vi "Plane.SetLongitude.vi"(8 "error in (no error)":errorcluster, 10 "SetLongitude":T1, 11 "Plane":refnum<class "Plane.lvclass">) -> (0 "error out":errorcluster, 3 "Plane out":refnum<class "Plane.lvclass">)   [LabVIEW 2020, in "Plane.lvclass"]
doc: "---------------------------------------------------------------\nJKI State Machine Objects™\nhttp://jki.net/state-machine-objects/\nCopyright (C) 2005-2015, JKI <info@jki.net>\nALL RIGHTS RESERVEDJKI State Machine Objects (SMO) 1.0.0.4\nJKI - JKI\nCopyright (c) 2015, JKI"
uses:
  Plane.lvclass
  Plane.lvclass/Plane.ctl
  Typedefs/PrivateEvents--Plane.SetLongitude.ctl
panel:
  # "For instructions on how to use the JKI State Machine Objects, examples and video tutorials, visit:\nhttp://jki.net/state-machine-objects/\n\nJKI State Machine Objects™\nhttp://jki.net/state-machine-objects/\nCopyright (C) 2005-2015, JKI <info@jki.net>\nALL RIGHTS RESERVED"
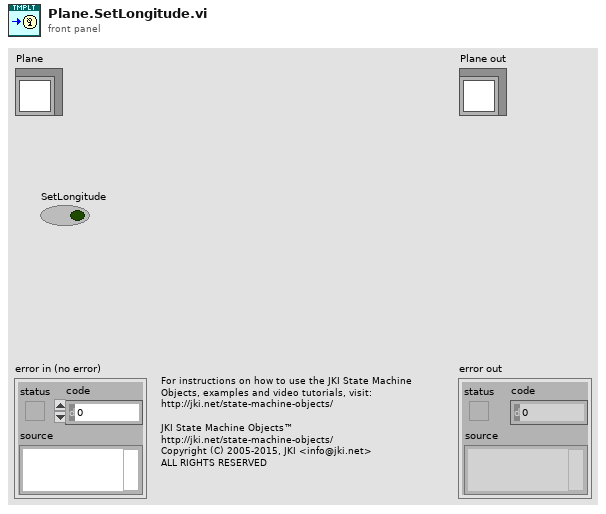
[diagram p1: front panel]
types:
  T1 = typedef "Plane.lvclass/PrivateEvents--Plane.SetLongitude.ctl" = bool
  T2 = typedef "Plane.lvclass/PrivateData--Ref.ctl" = refnum<data-value>
  T3 = typedef "Plane.lvclass/PrivateData--Cluster.ctl" = cluster{"Configuration":T4, "Public Events":T5, "Protected Events":T6, "Data":string, "Private Events":T7}
  T4 = typedef "Plane.lvclass/Configuration--Cluster.ctl" = cluster{"Suffix":string}
  T5 = typedef "Plane.lvclass/PublicEvents--Cluster.ctl" = cluster{"Data Changed":refnum<user-event>}
  T6 = typedef "Plane.lvclass/ProtectedEvents--Cluster.ctl" = cluster{"API_Template":refnum<user-event>}
  T7 = typedef "Plane.lvclass/PrivateEvents--Cluster.ctl" = cluster{"SetLatitude":refnum<user-event>, "SetLongitude":refnum<user-event>, "SetCoord":refnum<user-event>, "SetAltitude":refnum<user-event>, "SetHeading":refnum<user-event>, "SetSpeed":refnum<user-event>, "SetICAO":refnum<user-event>, "SetHDG":refnum<user-event>, "GetPlaneData":refnum<user-event>, "SetUpdateTime":refnum<user-event>}
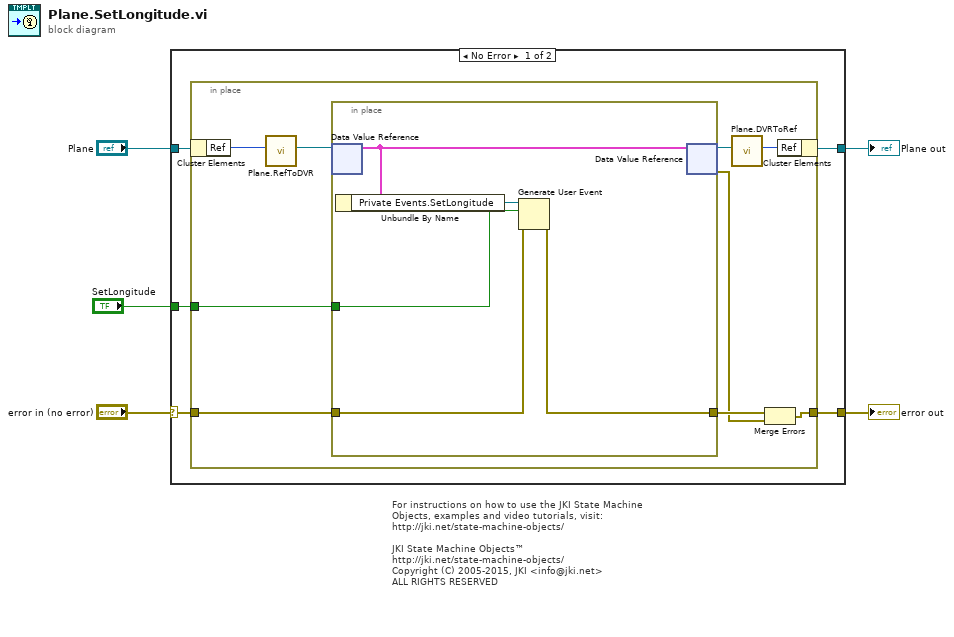
[diagram p0: block diagram]
diagram:
  # "For instructions on how to use the JKI State Machine Objects, examples and video tutorials, visit:\nhttp://jki.net/state-machine-objects/\n\nJKI State Machine Objects™\nhttp://jki.net/state-machine-objects/\nCopyright (C) 2005-2015, JKI <info@jki.net>\nALL RIGHTS RESERVED"
  n1 = case shown="No Error" "error in (no error)" {
    selector: "error in (no error)" -> [w8 w26]
    tunnel: [w7 w26] -> w4
    tunnel: [w9 w25] -> w5
    tunnel: "Plane" -> [w10 w25]
    tunnel: "SetLongitude" -> [w6 _]
    frame No Error {
      n2 = in-place {
        in-place-border: w8 -> [w19]
        in-place-border: [w16] -> w7
        in-place-border: w6 -> [w13]
        n3 = in-place-cluster #1(w10) -> ("Ref"=w15:u32)
        n4 = call "Plane.RefToDVR.vi"("Ref"=w15) -> ("Ref"=w12:T2)  [unwired: 10 in]
        n5 = in-place {
          in-place-border: w19 -> [w22]
          in-place-border: [w21] -> w18
          in-place-border: w13 -> [w20]
          n6 = in-place-dvr #2(w12) -> (w24:T3)  [unwired: 1 out]
          n7 = Unbundle By Name(w24) -> ("Private Events.SetLongitude"=w23:refnum<user-event>)
          n8 = Generate User Event(user event=w23, event data cluster=w20, error in=w22) -> (error out=w21:errorcluster)  [unwired: 1 in, 1 out]
          n9 = in-place-dvr #2(w24) -> (w14:T2, w17:errorcluster)
        }
        n10 = call "Plane.DVRToRef.vi"("Ref"=w14) -> ("Ref"=w11:u32)  [unwired: 10 in]
        n11 = Merge Errors(w18, w17) -> (w16:errorcluster)
        n12 = in-place-cluster #1("Ref"=w11) -> (w9:refnum<class "Plane.lvclass">)
      }
    }
    frame Error {
    }
  }
  "error out" <- w4
  "Plane out" <- w5
